vi "Query Trigger Mode.vi"(8 "error in (no error)":errorcluster, 11 "VISA resource name":refnum<visa-resource-name>) -> (0 "error out":errorcluster, 2 "trigger mode":T1 items=["Single", "Continuous", "Gated", "Burst"], 3 "VISA resource name out":refnum<visa-resource-name>)   [LabVIEW 2019, in "Pulse Rider PG-1000.lvlib"]
doc: "Query the instrument trigger source.\nThe trigger mode can be : gated, single, burst, continuous"
uses:
  <instrlib>/Pulse Rider PG-1000/Pulse Rider PG-1000.lvlib
  <instrlib>/Pulse Rider PG-1000/Public/Configure/Trigger/Trigger Mode.ctl
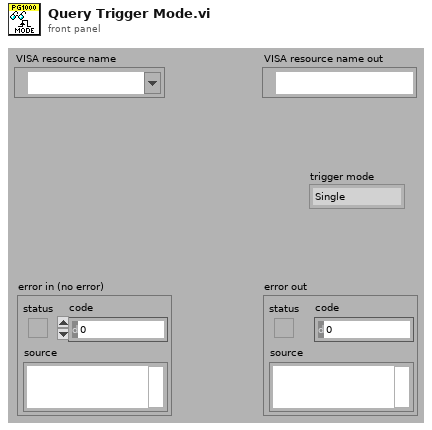
[diagram p1: front panel]
types:
  T1 = typedef "Pulse Rider PG-1000.lvlib/Trigger Mode.ctl" = u16
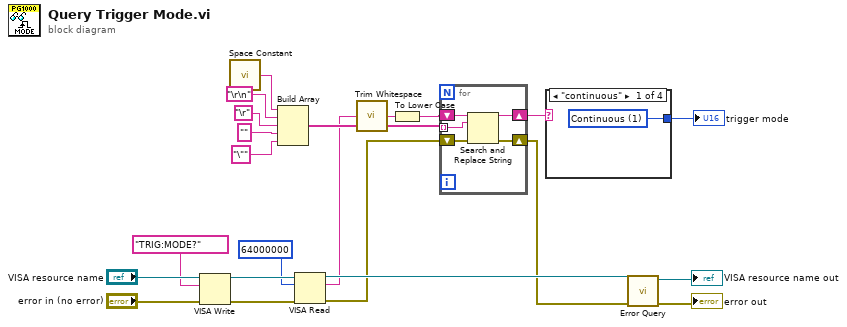
[diagram p0: block diagram]
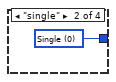
[diagram p2: hidden frame]
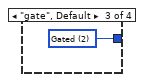
[diagram p3: hidden frame]
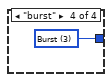
[diagram p4: hidden frame]
diagram:
  n1 = VISA Write(VISA resource name="VISA resource name", write buffer="TRIG:MODE?", error in (no error)="error in (no error)") -> (VISA resource name out=w18:refnum<visa-resource-name>, error out=w17:errorcluster)  [unwired: 1 out]
  n2 = call <vilib>:"Space Constant.vi"() -> ("String"=w12:string)
  n3 = Build Array(w12, "\r\n", "\r", "", "\"") -> (w7:string[])
  n4 = VISA Read(VISA resource name=w18, byte count=u32 64000000, error in (no error)=w17) -> (VISA resource name out=w15:refnum<visa-resource-name>, read buffer=w5:string, error out=w2:errorcluster)  [unwired: 1 out]
  n5 = call <vilib>:"Trim Whitespace.vi"("string"=w5) -> ("trimmed string"=w6:string)  [unwired: 1 in]
  n6 = To Lower Case(string=w6) -> (all lower case string=w4:string)
  n7 = for {
    tunnel: w7 -> [w25] mode=indexing
    shift-right: [w27] -> w13
    shift-left: w4 -> [w26]
    shift-right: [w23] -> w1
    shift-left: w2 -> [w24]
    n8 = Search and Replace String(input string=w26, search string=w25, error in=w24) -> (result string=w27:string, error out=w23:errorcluster)  [unwired: 5 in, 2 out]
  }
  n9 = case shown="\"continuous\"" w13 {
    tunnel: [w28 w29 w30 w31] -> w3
    frame "continuous" {
      w28 = T1 1 items=["Single", "Continuous", "Gated", "Burst"] ("trigger mode")
    }
    frame "single" {
      w29 = T1 0 items=["Single", "Continuous", "Gated", "Burst"] ("trigger mode")
    }
    frame "gate", Default {
      w30 = T1 2 items=["Single", "Continuous", "Gated", "Burst"] ("trigger mode")
    }
    frame "burst" {
      w31 = T1 3 items=["Single", "Continuous", "Gated", "Burst"] ("trigger mode")
    }
  }
  "trigger mode" <- w3
  n10 = call <instrlib>:"Error Query.vi"("error in (no error)"=w1, "VISA resource name"=w15) -> ("error out"=→"error out":errorcluster, "VISA resource name out"=→"VISA resource name out":refnum<visa-resource-name>)  [unwired: 6 in, 2 out]
